vi "dfd_FXPMath Delay Holder.vi"() -> ()   [LabVIEW 2017, in "NI_DigFilter_CodeGen.lvlib"]
uses:
  <vilib>/addons/Digital Filter Design/NI_DigFilter_CodeGen.lvlib
  <vilib>/rvi/FXPMathLib/basic elements/FxpDiscreteDelay/XNode/nifxpmath_DiscreteDelay.xnode
panel:
  out "Q":bool
  in  "D":bool
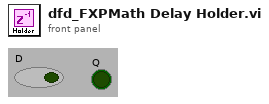
[diagram p1: front panel]
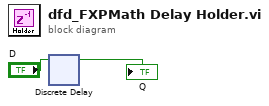
[diagram p0: block diagram]
diagram:
  n1 = xnode "Discrete Delay"("D"="D") -> ("Q"=→"Q":bool)
